vi "Graph_MaxMin_v00.vi"(8 "Reset MaxMin?":T2, 9 "Min (-1)":T3, 10 "Max (-1)":T4, 11 "Graph Errors":T1) -> (0 "Max":T4, 3 "Min":T3)   [LabVIEW 2010]
uses:
  Strict Type Defs/Graph Max.ctl
  Strict Type Defs/Graph Min.ctl
  Strict Type Defs/Graph Reset MaxMin.ctl
  Strict Type Defs/Graph Errors.ctl
panel:
  in  "Min typedef":T3
  in  "Max typedef":T4
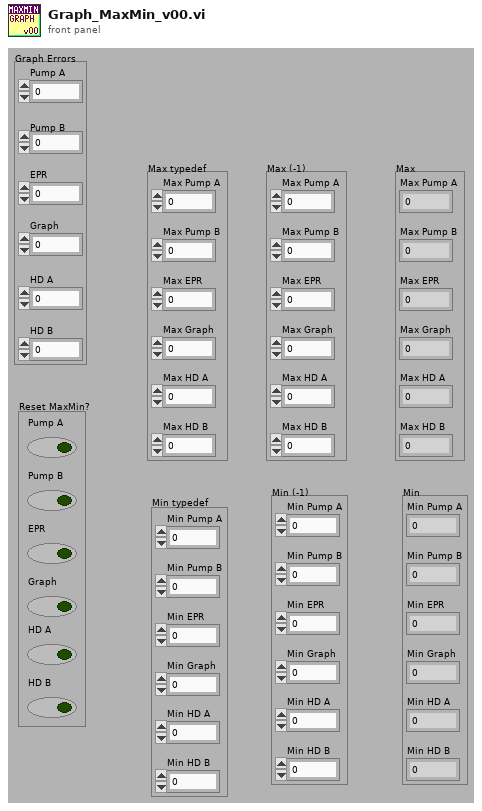
[diagram p1: front panel]
types:
  T1 = typedef "Graph Errors.ctl" = cluster{"Pump A":i16, "Pump B":i16, "EPR":i16, "Graph":i16, "HD A":i16, "HD B":i16}
  T2 = typedef "Graph Reset MaxMin.ctl" = cluster{"Pump A":bool, "Pump B":bool, "EPR":bool, "Graph":bool, "HD A":bool, "HD B":bool}
  T3 = typedef "Graph Min.ctl" = cluster{"Min Pump A":i16, "Min Pump B":i16, "Min EPR":i16, "Min Graph":i16, "Min HD A":i16, "Min HD B":i16}
  T4 = typedef "Graph Max.ctl" = cluster{"Max Pump A":i16, "Max Pump B":i16, "Max EPR":i16, "Max Graph":i16, "Max HD A":i16, "Max HD B":i16}
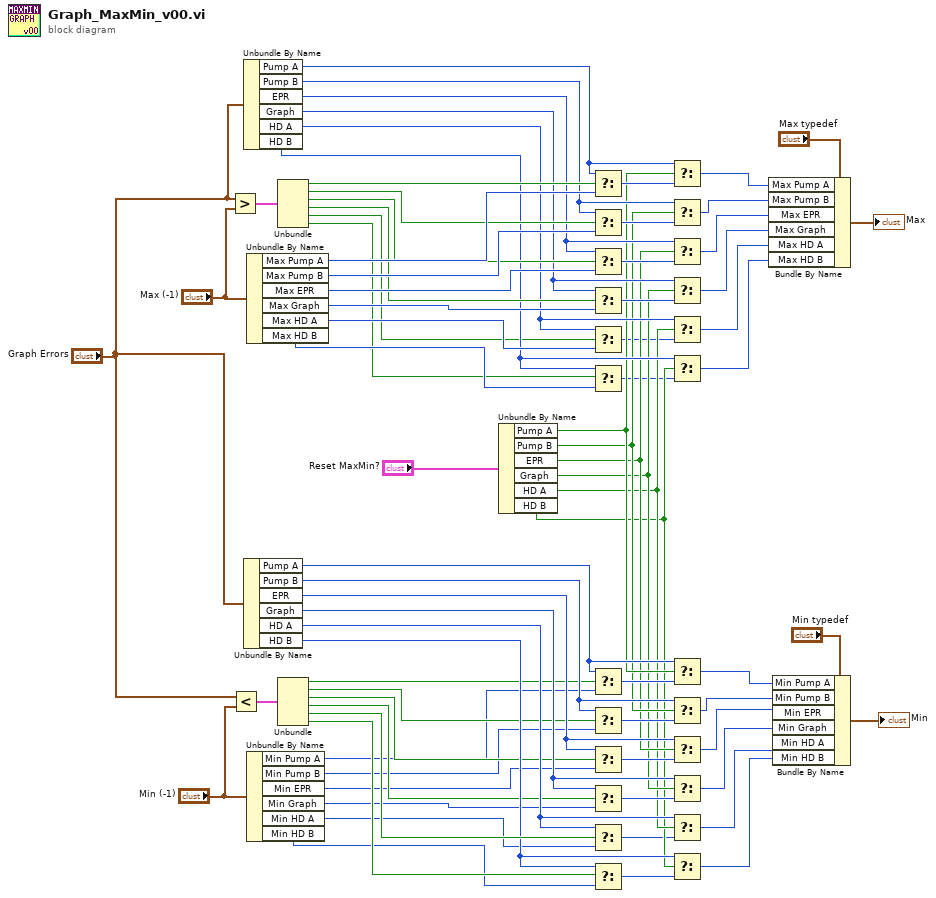
[diagram p0: block diagram]
diagram:
  n1 = Greater?(x="Graph Errors", y="Max (-1)") -> (0:w67:cluster{bool, bool, bool, bool, bool, bool})
  n2 = Less?(x="Graph Errors", y="Min (-1)") -> (x < y?=w18:cluster{bool, bool, bool, bool, bool, bool})
  n3 = Unbundle By Name("Graph Errors") -> ("Pump A"=w58:i16, "Pump B"=w57:i16, "EPR"=w56:i16, "Graph"=w55:i16, "HD A"=w47:i16, "HD B"=w46:i16)
  n4 = Unbundle By Name("Graph Errors") -> ("Pump A"=w32:i16, "Pump B"=w33:i16, "EPR"=w34:i16, "Graph"=w35:i16, "HD A"=w38:i16, "HD B"=w39:i16)
  n5 = Unbundle By Name("Max (-1)") -> ("Max Pump A"=w76:i16, "Max Pump B"=w75:i16, "Max EPR"=w74:i16, "Max Graph"=w73:i16, "Max HD A"=w48:i16, "Max HD B"=w49:i16)
  n6 = Unbundle By Name("Min (-1)") -> ("Min Pump A"=w20:i16, "Min Pump B"=w21:i16, "Min EPR"=w22:i16, "Min Graph"=w23:i16, "Min HD A"=w37:i16, "Min HD B"=w36:i16)
  n7 = Unbundle(w67) -> (w66:bool, w65:bool, w64:bool, w63:bool, w45:bool, w44:bool)
  n8 = Unbundle(w18) -> (w24:bool, w25:bool, w26:bool, w27:bool, w40:bool, w41:bool)
  n9 = Unbundle By Name("Reset MaxMin?") -> ("Pump A"=w16:bool, "Pump B"=w15:bool, "EPR"=w14:bool, "Graph"=w13:bool, "HD A"=w12:bool, "HD B"=w11:bool)
  n10 = Select(t=w58, s=w66, f=w76) -> (s? t:f=w59:i16)
  n11 = Select(t=w57, s=w65, f=w75) -> (s? t:f=w60:i16)
  n12 = Select(t=w56, s=w64, f=w74) -> (s? t:f=w61:i16)
  n13 = Select(t=w55, s=w63, f=w73) -> (s? t:f=w62:i16)
  n14 = Select(t=w47, s=w45, f=w48) -> (s? t:f=w1:i16)
  n15 = Select(t=w46, s=w44, f=w49) -> (s? t:f=w2:i16)
  n16 = Select(t=w32, s=w24, f=w20) -> (s? t:f=w31:i16)
  n17 = Select(t=w33, s=w25, f=w21) -> (s? t:f=w30:i16)
  n18 = Select(t=w34, s=w26, f=w22) -> (s? t:f=w29:i16)
  n19 = Select(t=w35, s=w27, f=w23) -> (s? t:f=w28:i16)
  n20 = Select(t=w38, s=w40, f=w37) -> (s? t:f=w4:i16)
  n21 = Select(t=w39, s=w41, f=w36) -> (s? t:f=w3:i16)
  n22 = Select(t=w58, s=w16, f=w59) -> (s? t:f=w50:i16)
  n23 = Select(t=w57, s=w15, f=w60) -> (s? t:f=w51:i16)
  n24 = Select(t=w56, s=w14, f=w61) -> (s? t:f=w52:i16)
  n25 = Select(t=w55, s=w13, f=w62) -> (s? t:f=w53:i16)
  n26 = Select(t=w47, s=w12, f=w1) -> (s? t:f=w43:i16)
  n27 = Select(t=w46, s=w11, f=w2) -> (s? t:f=w42:i16)
  n28 = Select(t=w32, s=w16, f=w31) -> (s? t:f=w10:i16)
  n29 = Select(t=w33, s=w15, f=w30) -> (s? t:f=w9:i16)
  n30 = Select(t=w34, s=w14, f=w29) -> (s? t:f=w8:i16)
  n31 = Select(t=w35, s=w13, f=w28) -> (s? t:f=w7:i16)
  n32 = Select(t=w38, s=w12, f=w4) -> (s? t:f=w6:i16)
  n33 = Select(t=w39, s=w11, f=w3) -> (s? t:f=w5:i16)
  n34 = Bundle By Name(cluster="Max typedef", "Max Pump A"=w50, "Max Pump B"=w51, "Max EPR"=w52, "Max Graph"=w53, "Max HD A"=w43, "Max HD B"=w42) -> (→"Max":T4)
  n35 = Bundle By Name(cluster="Min typedef", "Min Pump A"=w10, "Min Pump B"=w9, "Min EPR"=w8, "Min Graph"=w7, "Min HD A"=w6, "Min HD B"=w5) -> (→"Min":T3)
